vi "Test2.vi"() -> ()   [LabVIEW 2009]
panel:
  in  "FPGA IP Address":string
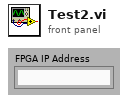
[diagram p1: front panel]
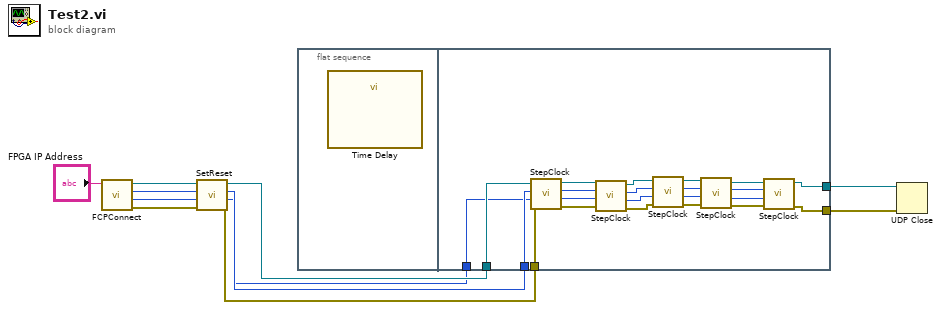
[diagram p0: block diagram]
diagram:
  n1 = call "FCPConnect.vi"("FPGA IP Address"="FPGA IP Address") -> ("error out"=w9:errorcluster, "Sequence Number"=w7:i32, "FPGA IP Address Out"=w8:u32, "connection ID out"=w10:refnum<k16>)  [unwired: 7 in]
  n2 = call "SetReset.vi"("error in (no error)"=w9, "SequenceNumber"=w7, "address"=w8, "connection ID"=w10) -> ("error out"=w3:errorcluster, "SequenceNumber out"=w4:i32, "Address out"=w5:u32, "connection ID out"=w6:refnum<k16>)  [unwired: 4 in]
  n3 = flat-sequence {
    tunnel: w6 -> [w33]
    tunnel: w5 -> [w32]
    tunnel: w4 -> [w31]
    tunnel: w3 -> [w30]
    tunnel: [w13] -> w2
    tunnel: [w12] -> w1
    frame #0 {
      n4 = call "Time Delay"() -> ()  [unwired: 11 in, 1 out]
    }
    frame #1 {
      n5 = call "StepClock.vi"("error in (no error)"=w30, "SequenceNumber"=w31, "address"=w32, "connection ID"=w33) -> ("error out"=w26:errorcluster, "SequenceNumber out"=w27:i32, "address out"=w28:u32, "connection ID out"=w29:refnum<k16>)  [unwired: 4 in]
      n6 = call "StepClock.vi"("error in (no error)"=w26, "SequenceNumber"=w27, "address"=w28, "connection ID"=w29) -> ("error out"=w22:errorcluster, "SequenceNumber out"=w23:i32, "address out"=w24:u32, "connection ID out"=w25:refnum<k16>)  [unwired: 4 in]
      n7 = call "StepClock.vi"("error in (no error)"=w22, "SequenceNumber"=w23, "address"=w24, "connection ID"=w25) -> ("error out"=w18:errorcluster, "SequenceNumber out"=w19:i32, "address out"=w20:u32, "connection ID out"=w21:refnum<k16>)  [unwired: 4 in]
      n8 = call "StepClock.vi"("error in (no error)"=w18, "SequenceNumber"=w19, "address"=w20, "connection ID"=w21) -> ("error out"=w17:errorcluster, "SequenceNumber out"=w16:i32, "address out"=w15:u32, "connection ID out"=w14:refnum<k16>)  [unwired: 4 in]
      n9 = call "StepClock.vi"("error in (no error)"=w17, "SequenceNumber"=w16, "address"=w15, "connection ID"=w14) -> ("error out"=w12:errorcluster, "connection ID out"=w13:refnum<k16>)  [unwired: 4 in, 2 out]
    }
  }
  n10 = UDP Close(connection ID=w2, 8:w1) -> ()  [unwired: 2 out]
